vi "S4GUI_001.vi"() -> ()   [LabVIEW 2018] (continued)
                    n596 = stacked-sequence "Atualizacao dos indicadores inferiores do CANAL C da tela principal" {
                      tunnel: w1340 -> [w1355 w1358 w1363 w1372 w1375 w1379]
                      tunnel: [w1341 _ _ _ _ _] -> w1339
                      tunnel: [_ w1356 _ _ _ _] -> w1338
                      tunnel: [_ _ w1361 _ _ _] -> w1337
                      tunnel: [_ _ _ w1366 _ _] -> w1336
                      tunnel: [_ _ _ _ w1373 _] -> w1335
                      tunnel: [_ _ _ _ _ w1376] -> w1334
                      frame #0 {
                        # "SubImage"
                        n597 = Unbundle By Name(w1355) -> ("INITIAL_LINE"=w1353:u16, "FINAL_LINE"=w1352:u16, "INITIAL_COLUMN"=w1351:u16, "FINAL_COLUMN"=w1350:u16)
                        n598 = Number To Decimal String(number=w1353) -> (decimal integer string=w1349:string)  [unwired: 1 in]
                        n599 = Number To Decimal String(number=w1352) -> (decimal integer string=w1347:string)  [unwired: 1 in]
                        n600 = Number To Decimal String(number=w1351) -> (decimal integer string=w1345:string)  [unwired: 1 in]
                        n601 = Number To Decimal String(number=w1350) -> (decimal integer string=w1343:string)  [unwired: 1 in]
                        n602 = Concatenate Strings("[", w1349, ":", w1347, ",", w1345, ":", w1343, "]") -> (w1341:string)
                      }
                      frame #1 {
                        # "Em Active"
                        n603 = Unbundle By Name(w1358) -> ("EM_MODE"=w1357:u8)
                        n604 = case shown="0, Default" w1357 {
                          tunnel: ["Electron M." ("EmActive1") "Convent." ("EmActive1")] -> w1356
                          frame 0, Default {
                          }
                          frame 1 {
                          }
                        }
                      }
                      frame #2 {
                        # "Pre Amp"
                        n605 = Unbundle By Name(w1363) -> ("PREAMP"=w1362:u8)
                        n606 = case shown="1" w1362 {
                          tunnel: ["Gain 1" ("EmActive1") "Gain 2" ("EmActive1")] -> w1361
                          frame 0, Default {
                          }
                          frame 1 {
                          }
                        }
                      }
                      frame #3 {
                        # "Binning"
                        n607 = Unbundle By Name(w1372) -> ("VBIN"=w1371:u16, "HBIN"=w1370:u16)
                        n608 = Number To Decimal String(number=w1370) -> (decimal integer string=w1367:string)  [unwired: 1 in]
                        n609 = Number To Decimal String(number=w1371) -> (decimal integer string=w1369:string)  [unwired: 1 in]
                        n610 = Concatenate Strings(w1369, "x", w1367) -> (w1366:string)
                      }
                      frame #4 {
                        # "Gain"
                        n611 = Unbundle By Name(w1375) -> ("EM_GAIN"=w1374:u16)
                        n612 = Number To Decimal String(number=w1374) -> (decimal integer string=w1373:string)  [unwired: 1 in]
                      }
                      frame #5 {
                        # "Readout"
                        n613 = Unbundle By Name(w1379) -> ("EM_MODE"=w1378:u8, "READOUT_RATE"=w1377:u8)
                        n614 = case shown="0, Default" w1378 {
                          tunnel: w1377 -> [w1381 w1387]
                          tunnel: [w1380 w1386] -> w1376
                          frame 0, Default {
                            n615 = case shown="0, Default" w1381 {
                              tunnel: ["30 MHz" ("EmActive1") "20 MHz" ("EmActive1") "10 MHz" ("EmActive1") "1 MHz" ("EmActive1")] -> w1380
                              frame 0, Default {
                              }
                              frame 1 {
                              }
                              frame 2 {
                              }
                              frame 3 {
                              }
                            }
                          }
                          frame 1 {
                            n616 = case shown="1" w1387 {
                              tunnel: ["1 MHz" ("EmActive1") "0.1 MHz" ("EmActive1")] -> w1386
                              frame 0, Default {
                              }
                              frame 1 {
                              }
                            }
                          }
                        }
                      }
                    }
                  }
                }
                n617 = Unbundle By Name(w1264) -> ("INITIAL_LINE"=w1269:u16, "INITIAL_COLUMN"=w1267:u16, "FINAL_LINE"=w1270:u16, "FINAL_COLUMN"=w1268:u16, "VBIN"=w1273:u16, "HBIN"=w1329:u16, "PREAMP"=w1272:u8, "EM_GAIN"=w1271:u16, "READOUT_RATE"=w1266:u8, "SHUTTER_OPENNING_TIME"=w1328:u16, "SHUTTER_CLOSING_TIME"=w1327:u16, "VERTICAL_SHIFT_SPEED"=w1326:u8, "READ_MODE"=w1325:u8, "VERTICAL_CLOCK_VOLTAGE"=w1324:u8, "AD_CHANNEL"=w1323:u32, "SHUTTER_MODE"=w1318:u8, "SHUTTER_TTL"=w1319:u8, "TRIGGER_MODE"=w1320:u8, "FRAME_TRANSFER"=w1321:bool, "ACQUISITION_MODE"=w1322:u8, "EM_MODE"=w1265:u8)
                n618 = Not(x=w1292) -> (.not. x?=w1312:bool)
                n619 = Not(x=w1291) -> (.not. x?=w1310:bool)
                n620 = Not(x=w1290) -> (.not. x?=w1311:bool)
                n621 = Not(x=w1289) -> (.not. x?=w1309:bool)
                n622 = Not(x=w1295) -> (.not. x?=w1314:bool)
                n623 = Not(x=w1294) -> (.not. x?=w1313:bool)
                n624 = Not(x=w1293) -> (.not. x?=w1315:bool)
                n625 = property on="Image FInal Column 3" class="DigNum (strict)"("Blinking"=w1312) -> ()  [unwired: 2 in, 2 out]
                n626 = property on="Frame Transfer 3" class="Bool (strict)"("Blinking"=w1310) -> ()  [unwired: 2 in, 2 out]
                n627 = property on="Vertical Clock Voltage 3" class="Ring (strict)"("Blinking"=w1311) -> ()  [unwired: 2 in, 2 out]
                n628 = property on="A/D Channel 3" class="DigNum (strict)"("Blinking"=w1309) -> ()  [unwired: 2 in, 2 out]
                n629 = property on="Image Initial Line 3" class="DigNum (strict)"("Blinking"=w1314) -> ()  [unwired: 2 in, 2 out]
                n630 = property on="Image Initial Column 3" class="DigNum (strict)"("Blinking"=w1313) -> ()  [unwired: 2 in, 2 out]
                n631 = property on="Image Final Line 3" class="DigNum (strict)"("Blinking"=w1315) -> ()  [unwired: 2 in, 2 out]
                n632 = Not(x=w1284) -> (.not. x?=w1305:bool)
                n633 = Not(x=w1283) -> (.not. x?=w1307:bool)
                n634 = Not(x=w1282) -> (.not. x?=w1306:bool)
                n635 = Not(x=w1281) -> (.not. x?=w1308:bool)
                n636 = Not(x=w1288) -> (.not. x?=w1304:bool)
                n637 = Not(x=w1287) -> (.not. x?=w1286:bool)
                n638 = Not(x=w1285) -> (.not. x?=w1303:bool)
                n639 = property on="Shutter Openning Time 3" class="DigNum (strict)"("Blinking"=w1305) -> ()  [unwired: 2 in, 2 out]
                n640 = property on="Shutter Closing Time 3" class="DigNum (strict)"("Blinking"=w1307) -> ()  [unwired: 2 in, 2 out]
                n641 = property on="Vertical Binning 3" class="DigNum (strict)"("Blinking"=w1306) -> ()  [unwired: 2 in, 2 out]
                n642 = property on="Horizontal Binning 3" class="DigNum (strict)"("Blinking"=w1308) -> ()  [unwired: 2 in, 2 out]
                n643 = property on="CCD EM Gain 3" class="DigNum (strict)"("Blinking"=w1304) -> ()  [unwired: 2 in, 2 out]
                n644 = property on="Shutter Mode 3" class="Ring (strict)"("Blinking"=w1286) -> ()  [unwired: 2 in, 2 out]
                n645 = property on="Shutter TTL 3" class="Ring (strict)"("Blinking"=w1303) -> ()  [unwired: 2 in, 2 out]
                n646 = local read "Cameras Cluster"() -> (w1331:T5)
                n647 = Bundle By Name(cluster=w1331, "Current Configuration.Image Initial Line 3"=w1269, "Current Configuration.Image Initial Column 3"=w1267, "Current Configuration.Image Final Line 3"=w1270, "Current Configuration.Image FInal Column 3"=w1268, "Current Configuration.Vertical Binning 3"=w1273, "Current Configuration.Horizontal Binning 3"=w1329, "Current Configuration.Pre-amplification Gain 3"=w1272, "Current Configuration.CCD EM Gain 3"=w1271, "Current Configuration.Readout Rate 3"=w1266, "Current Configuration.Shutter Openning Time 3"=w1328, "Current Configuration.Shutter Closing Time 3"=w1327, "Current Configuration.Vertical Shift Speed 3"=w1326, "Current Configuration.Read Mode 3"=w1325, "Current Configuration.Vertical Clock Voltage 3"=w1324, "Current Configuration.A/D Channel 3"=w1323, "Current Configuration.Shutter Mode 3"=w1318, "Current Configuration.Shutter TTL 3"=w1319, "Current Configuration.Trigger Mode 3"=w1320, "Current Configuration.Frame Transfer 3"=w1321, "Current Configuration.Acquisition Mode 3"=w1322, "Current Configuration.CCD EM Mode 3"=w1265) -> (w1330:T5)
                n648 = Not(x=w1280) -> (.not. x?=w1296:bool)
                n649 = Not(x=w1276) -> (.not. x?=w1299:bool)
                n650 = Not(x=w1275) -> (.not. x?=w1297:bool)
                n651 = Not(x=w1274) -> (.not. x?=w1298:bool)
                n652 = Not(x=w1279) -> (.not. x?=w1301:bool)
                n653 = Not(x=w1278) -> (.not. x?=w1300:bool)
                n654 = Not(x=w1277) -> (.not. x?=w1302:bool)
                n655 = local write "RO3"(w1258) -> ()
                n656 = local write "B3"(w1260) -> ()
                n657 = local write "PA3"(w1261) -> ()
                n658 = local write "EA3"(w1262) -> ()
                n659 = local write "G3"(w1259) -> ()
                n660 = local write "SI3"(w1263) -> ()
                n661 = property on="Acquisition Mode 3" class="Ring (strict)"("Blinking"=w1296) -> ()  [unwired: 2 in, 2 out]
                n662 = property on="Readout Rate 3" class="Ring (strict)"("Blinking"=w1299) -> ()  [unwired: 2 in, 2 out]
                n663 = property on="Vertical Shift Speed 3" class="Ring (strict)"("Blinking"=w1297) -> ()  [unwired: 2 in, 2 out]
                n664 = property on="CCD EM Mode 3" class="Ring (strict)"("Blinking"=w1298) -> ()  [unwired: 2 in, 2 out]
                n665 = property on="Trigger Mode 3" class="Ring (strict)"("Blinking"=w1301) -> ()  [unwired: 2 in, 2 out]
                n666 = property on="Read Mode 3" class="Ring (strict)"("Blinking"=w1300) -> ()  [unwired: 2 in, 2 out]
                n667 = property on="Pre-amplification Gain 3" class="Ring (strict)"("Blinking"=w1302) -> ()  [unwired: 2 in, 2 out]
                n668 = local write "Cameras Cluster"(w1330) -> ()
                n669 = Compound Arithmetic op=AND(w1280, w1279, w1278, w1277, w1276, w1275, w1274, w1288, w1287, w1285, w1284, w1283, w1282, w1281, w1295, w1294, w1293, w1292, w1291, w1290, w1289) -> (→"CCD checked 3":bool)
              }
              frame #18 {
                # "Carrega coluna do Channel 4"
                # "Aba:  Eng->Camera"
                n670 = Unbundle By Name(w1465) -> ("ChannelD_CCD"=w1397:T21, "CHD_Checked Params"=w1450:T22, "ChannelD_Status.connection"=w1396:bool)
                n671 = Unbundle By Name(w1450) -> ("ACQUISITION_MODE"=w1414:bool, "TRIGGER_MODE"=w1413:bool, "READ_MODE"=w1412:bool, "PREAMP"=w1410:bool, "READOUT_RATE"=w1409:bool, "VERTICAL_SHIFT_SPEED"=w1408:bool, "EM_MODE"=w1407:bool, "EM_GAIN"=w1421:bool, "SHUTTER_MODE"=w1420:bool, "SHUTTER_TTL"=w1419:bool, "SHUTTER_OPENING_TIME"=w1418:bool, "SHUTTER_CLOSING_TIME"=w1417:bool, "VBIN"=w1416:bool, "HBIN"=w1415:bool, "INITIAL_LINE"=w1428:bool, "INITIAL_COLUMN"=w1427:bool, "FINAL_LINE"=w1426:bool, "FINAL_COLUMN"=w1425:bool, "FRAME_TRANSFER"=w1424:bool, "VERTICAL_CLOCK_VOLTAGE"=w1423:bool, "AD_CHANNEL"=w1422:bool)
                n672 = case shown="False" w1396 {
                  tunnel: w1397 -> [_ w1473]
                  tunnel: [w1466 w1472] -> w1395
                  tunnel: [w1466 w1471] -> w1394
                  tunnel: [w1466 w1470] -> w1393
                  tunnel: [w1466 w1469] -> w1392
                  tunnel: [w1466 w1468] -> w1391
                  tunnel: [w1466 w1467] -> w1390
                  frame False {
                    w1466 = ""
                  }
                  frame True {
                    n673 = stacked-sequence "Atualizacao dos indicadores inferiores do CANAL D da tela principal" {
                      tunnel: w1473 -> [w1488 w1491 w1496 w1505 w1508 w1512]
                      tunnel: [w1474 _ _ _ _ _] -> w1472
                      tunnel: [_ w1489 _ _ _ _] -> w1471
                      tunnel: [_ _ w1494 _ _ _] -> w1470
                      tunnel: [_ _ _ w1499 _ _] -> w1469
                      tunnel: [_ _ _ _ w1506 _] -> w1468
                      tunnel: [_ _ _ _ _ w1509] -> w1467
                      frame #0 {
                        # "SubImage"
                        n674 = Unbundle By Name(w1488) -> ("INITIAL_LINE"=w1486:u16, "FINAL_LINE"=w1485:u16, "INITIAL_COLUMN"=w1484:u16, "FINAL_COLUMN"=w1483:u16)
                        n675 = Number To Decimal String(number=w1486) -> (decimal integer string=w1482:string)  [unwired: 1 in]
                        n676 = Number To Decimal String(number=w1485) -> (decimal integer string=w1480:string)  [unwired: 1 in]
                        n677 = Number To Decimal String(number=w1484) -> (decimal integer string=w1478:string)  [unwired: 1 in]
                        n678 = Number To Decimal String(number=w1483) -> (decimal integer string=w1476:string)  [unwired: 1 in]
                        n679 = Concatenate Strings("[", w1482, ":", w1480, ",", w1478, ":", w1476, "]") -> (w1474:string)
                      }
                      frame #1 {
                        # "Em Active"
                        n680 = Unbundle By Name(w1491) -> ("EM_MODE"=w1490:u8)
                        n681 = case shown="0, Default" w1490 {
                          tunnel: ["Electron M." ("EmActive1") "Convent." ("EmActive1")] -> w1489
                          frame 0, Default {
                          }
                          frame 1 {
                          }
                        }
                      }
                      frame #2 {
                        # "Pre Amp"
                        n682 = Unbundle By Name(w1496) -> ("PREAMP"=w1495:u8)
                        n683 = case shown="1" w1495 {
                          tunnel: ["Gain 1" ("EmActive1") "Gain 2" ("EmActive1")] -> w1494
                          frame 0, Default {
                          }
                          frame 1 {
                          }
                        }
                      }
                      frame #3 {
                        # "Binning"
                        n684 = Unbundle By Name(w1505) -> ("VBIN"=w1504:u16, "HBIN"=w1503:u16)
                        n685 = Number To Decimal String(number=w1503) -> (decimal integer string=w1500:string)  [unwired: 1 in]
                        n686 = Number To Decimal String(number=w1504) -> (decimal integer string=w1502:string)  [unwired: 1 in]
                        n687 = Concatenate Strings(w1502, "x", w1500) -> (w1499:string)
                      }
                      frame #4 {
                        # "Gain"
                        n688 = Unbundle By Name(w1508) -> ("EM_GAIN"=w1507:u16)
                        n689 = Number To Decimal String(number=w1507) -> (decimal integer string=w1506:string)  [unwired: 1 in]
                      }
                      frame #5 {
                        # "Readout"
                        n690 = Unbundle By Name(w1512) -> ("EM_MODE"=w1511:u8, "READOUT_RATE"=w1510:u8)
                        n691 = case shown="0, Default" w1511 {
                          tunnel: w1510 -> [w1514 w1520]
                          tunnel: [w1513 w1519] -> w1509
                          frame 0, Default {
                            n692 = case shown="0, Default" w1514 {
                              tunnel: ["30 MHz" ("EmActive1") "20 MHz" ("EmActive1") "10 MHz" ("EmActive1") "1 MHz" ("EmActive1")] -> w1513
                              frame 0, Default {
                              }
                              frame 1 {
                              }
                              frame 2 {
                              }
                              frame 3 {
                              }
                            }
                          }
                          frame 1 {
                            n693 = case shown="1" w1520 {
                              tunnel: ["1 MHz" ("EmActive1") "0.1 MHz" ("EmActive1")] -> w1519
                              frame 0, Default {
                              }
                              frame 1 {
                              }
                            }
                          }
                        }
                      }
                    }
                  }
                }
                n694 = Unbundle By Name(w1397) -> ("INITIAL_LINE"=w1402:u16, "INITIAL_COLUMN"=w1400:u16, "FINAL_LINE"=w1403:u16, "FINAL_COLUMN"=w1401:u16, "VBIN"=w1406:u16, "HBIN"=w1462:u16, "PREAMP"=w1405:u8, "EM_GAIN"=w1404:u16, "READOUT_RATE"=w1399:u8, "SHUTTER_OPENNING_TIME"=w1461:u16, "SHUTTER_CLOSING_TIME"=w1460:u16, "VERTICAL_SHIFT_SPEED"=w1459:u8, "READ_MODE"=w1458:u8, "VERTICAL_CLOCK_VOLTAGE"=w1457:u8, "AD_CHANNEL"=w1456:u32, "SHUTTER_MODE"=w1451:u8, "SHUTTER_TTL"=w1452:u8, "TRIGGER_MODE"=w1453:u8, "FRAME_TRANSFER"=w1454:bool, "ACQUISITION_MODE"=w1455:u8, "EM_MODE"=w1398:u8)
                n695 = Not(x=w1425) -> (.not. x?=w1445:bool)
                n696 = Not(x=w1424) -> (.not. x?=w1443:bool)
                n697 = Not(x=w1423) -> (.not. x?=w1444:bool)
                n698 = Not(x=w1422) -> (.not. x?=w1442:bool)
                n699 = Not(x=w1428) -> (.not. x?=w1447:bool)
                n700 = Not(x=w1427) -> (.not. x?=w1446:bool)
                n701 = Not(x=w1426) -> (.not. x?=w1448:bool)
                n702 = property on="Image FInal Column 4" class="DigNum (strict)"("Blinking"=w1445) -> ()  [unwired: 2 in, 2 out]
                n703 = property on="Frame Transfer 4" class="Bool (strict)"("Blinking"=w1443) -> ()  [unwired: 2 in, 2 out]
                n704 = property on="Vertical Clock Voltage 4" class="Ring (strict)"("Blinking"=w1444) -> ()  [unwired: 2 in, 2 out]
                n705 = property on="A/D Channel 4" class="DigNum (strict)"("Blinking"=w1442) -> ()  [unwired: 2 in, 2 out]
                n706 = property on="Image Initial Line 4" class="DigNum (strict)"("Blinking"=w1447) -> ()  [unwired: 2 in, 2 out]
                n707 = property on="Image Initial Column 4" class="DigNum (strict)"("Blinking"=w1446) -> ()  [unwired: 2 in, 2 out]
                n708 = property on="Image Final Line 4" class="DigNum (strict)"("Blinking"=w1448) -> ()  [unwired: 2 in, 2 out]
                n709 = Not(x=w1418) -> (.not. x?=w1438:bool)
                n710 = Not(x=w1417) -> (.not. x?=w1440:bool)
                n711 = Not(x=w1416) -> (.not. x?=w1439:bool)
                n712 = Not(x=w1415) -> (.not. x?=w1441:bool)
                n713 = Not(x=w1421) -> (.not. x?=w1436:bool)
                n714 = Not(x=w1420) -> (.not. x?=w1437:bool)
                n715 = Not(x=w1419) -> (.not. x?=w1435:bool)
                n716 = property on="Shutter Openning Time 4" class="DigNum (strict)"("Blinking"=w1438) -> ()  [unwired: 2 in, 2 out]
                n717 = property on="Shutter Closing Time 4" class="DigNum (strict)"("Blinking"=w1440) -> ()  [unwired: 2 in, 2 out]
                n718 = property on="Vertical Binning 4" class="DigNum (strict)"("Blinking"=w1439) -> ()  [unwired: 2 in, 2 out]
                n719 = property on="Horizontal Binning 4" class="DigNum (strict)"("Blinking"=w1441) -> ()  [unwired: 2 in, 2 out]
                n720 = property on="CCD EM Gain 4" class="DigNum (strict)"("Blinking"=w1436) -> ()  [unwired: 2 in, 2 out]
                n721 = property on="Shutter Mode 4" class="Ring (strict)"("Blinking"=w1437) -> ()  [unwired: 2 in, 2 out]
                n722 = property on="Shutter TTL 4" class="Ring (strict)"("Blinking"=w1435) -> ()  [unwired: 2 in, 2 out]
                n723 = local read "Cameras Cluster"() -> (w1464:T5)
                n724 = Bundle By Name(cluster=w1464, "Current Configuration.Image Initial Line 4"=w1402, "Current Configuration.Image Initial Column 4"=w1400, "Current Configuration.Image Final Line 4"=w1403, "Current Configuration.Image FInal Column 4"=w1401, "Current Configuration.Vertical Binning 4"=w1406, "Current Configuration.Horizontal Binning 4"=w1462, "Current Configuration.Pre-amplification Gain 4"=w1405, "Current Configuration.CCD EM Gain 4"=w1404, "Current Configuration.Readout Rate 4"=w1399, "Current Configuration.Shutter Openning Time 4"=w1461, "Current Configuration.Shutter Closing Time 4"=w1460, "Current Configuration.Vertical Shift Speed 4"=w1459, "Current Configuration.Read Mode 4"=w1458, "Current Configuration.Vertical Clock Voltage 4"=w1457, "Current Configuration.A/D Channel 4"=w1456, "Current Configuration.Shutter Mode 4"=w1451, "Current Configuration.Shutter TTL 4"=w1452, "Current Configuration.Trigger Mode 4"=w1453, "Current Configuration.Frame Transfer 4"=w1454, "Current Configuration.Acquisition Mode 4"=w1455, "Current Configuration.CCD EM Mode 4"=w1398) -> (w1463:T5)
                n725 = local write "SI4"(w1395) -> ()
                n726 = local write "RO4"(w1390) -> ()
                n727 = local write "PA4"(w1393) -> ()
                n728 = local write "EA4"(w1394) -> ()
                n729 = local write "G4"(w1391) -> ()
                n730 = local write "B4"(w1392) -> ()
                n731 = Not(x=w1414) -> (.not. x?=w1429:bool)
                n732 = Not(x=w1409) -> (.not. x?=w1432:bool)
                n733 = Not(x=w1408) -> (.not. x?=w1430:bool)
                n734 = Not(x=w1407) -> (.not. x?=w1431:bool)
                n735 = Not(x=w1413) -> (.not. x?=w1433:bool)
                n736 = Not(x=w1412) -> (.not. x?=w1411:bool)
                n737 = Not(x=w1410) -> (.not. x?=w1434:bool)
                n738 = property on="Acquisition Mode 4" class="Ring (strict)"("Blinking"=w1429) -> ()  [unwired: 2 in, 2 out]
                n739 = property on="Readout Rate 4" class="Ring (strict)"("Blinking"=w1432) -> ()  [unwired: 2 in, 2 out]
                n740 = property on="Vertical Shift Speed 4" class="Ring (strict)"("Blinking"=w1430) -> ()  [unwired: 2 in, 2 out]
                n741 = property on="CCD EM Mode 4" class="Ring (strict)"("Blinking"=w1431) -> ()  [unwired: 2 in, 2 out]
                n742 = property on="Trigger Mode 4" class="Ring (strict)"("Blinking"=w1433) -> ()  [unwired: 2 in, 2 out]
                n743 = property on="Read Mode 4" class="Ring (strict)"("Blinking"=w1411) -> ()  [unwired: 2 in, 2 out]
                n744 = property on="Pre-amplification Gain 4" class="Ring (strict)"("Blinking"=w1434) -> ()  [unwired: 2 in, 2 out]
                n745 = local write "Cameras Cluster"(w1463) -> ()
                n746 = Compound Arithmetic op=AND(w1414, w1413, w1412, w1410, w1409, w1408, w1407, w1421, w1420, w1419, w1418, w1417, w1416, w1415, w1428, w1427, w1426, w1425, w1424, w1423, w1422) -> (→"CCD checked 4":bool)
              }
            }
            n747 = stacked-sequence {
              tunnel: w179 -> [w191 w195 w203 w210 w224]
              tunnel: w178 -> [w190 w194 w202 w209 w223]
              tunnel: [_ _ _ _ w215] -> w170
              tunnel: [_ _ _ _ w216] -> w169
              frame #0 {
                n748 = call-dynamic "Read AcquisitionA.vi"("error in (no error)"=w190, "S4ACS_GUI in"=w191) -> ("error out"=w187:errorcluster, "Acquisition.lvclass"=w189:refnum<class "Acquisition.lvclass">)  [unwired: 7 in, 1 out]
                n749 = call-dynamic "Read Channel.vi"("error in (no error)"=w187, "Acquisition in"=w189) -> ("error out"=w186:errorcluster, "Channel.lvclass"=w188:refnum<class "Channel.lvclass">)  [unwired: 7 in, 1 out]
                n750 = call-dynamic "Read CyclesDone.vi"("error in (no error)"=w186, "Channel in"=w188) -> ("error out"=→"error out 6":errorcluster, "CyclesDone"=→"Cycles Done ch1":u32)  [unwired: 7 in, 1 out]
              }
              frame #1 {
                n751 = call "Read AcquisitionB.vi"("error in (no error)"=w194, "S4ACS_GUI in"=w195) -> ("error out"=w197:errorcluster, "Acquisition.lvclass"=w198:refnum<class "Acquisition.lvclass">)  [unwired: 7 in, 1 out]
                n752 = call-dynamic "Read Channel.vi"("error in (no error)"=w197, "Acquisition in"=w198) -> ("error out"=w196:errorcluster, "Channel.lvclass"=w199:refnum<class "Channel.lvclass">)  [unwired: 7 in, 1 out]
                n753 = call-dynamic "Read CyclesDone.vi"("error in (no error)"=w196, "Channel in"=w199) -> ("error out"=→"error out 4":errorcluster, "CyclesDone"=→"Cycles Done ch2":u32)  [unwired: 7 in, 1 out]
              }
              frame #2 {
                n754 = call-dynamic "Read AcquisitionC.vi"("error in (no error)"=w202, "S4ACS_GUI in"=w203) -> ("error out"=w205:errorcluster, "Acquisition.lvclass"=w206:refnum<class "Acquisition.lvclass">)  [unwired: 7 in, 1 out]
                n755 = call-dynamic "Read Channel.vi"("error in (no error)"=w205, "Acquisition in"=w206) -> ("error out"=w204:errorcluster, "Channel.lvclass"=w207:refnum<class "Channel.lvclass">)  [unwired: 7 in, 1 out]
                n756 = call-dynamic "Read CyclesDone.vi"("error in (no error)"=w204, "Channel in"=w207) -> ("error out"=→"error out 5":errorcluster, "CyclesDone"=→"Cycles Done ch3":u32)  [unwired: 7 in, 1 out]
              }
              frame #3 {
                n757 = call-dynamic "Read AcquisitionD.vi"("error in (no error)"=w209, "S4ACS_GUI in"=w210) -> ("error out"=w212:errorcluster, "Acquisition.lvclass"=w213:refnum<class "Acquisition.lvclass">)  [unwired: 7 in, 1 out]
                n758 = call-dynamic "Read Channel.vi"("error in (no error)"=w212, "Acquisition in"=w213) -> ("error out"=w211:errorcluster, "Channel.lvclass"=w214:refnum<class "Channel.lvclass">)  [unwired: 7 in, 1 out]
                n759 = call-dynamic "Read CyclesDone.vi"("error in (no error)"=w211, "Channel in"=w214) -> ("CyclesDone"=→"Cycles Done ch4":u32)  [unwired: 7 in, 2 out]
              }
              frame #4 {
                (unwired) cluster{"AG status":bool, "rotator":dbl} {"AG status"=FALSE, "rotator"=0.0} ("element")
                n760 = call-dynamic "Read guider queue.vi"("error in (no error)"=w223, "S4GUI in"=w224) -> ("error out"=w218:errorcluster, "guider queue"=w222:refnum<queue>, "S4GUI out"=w217:refnum<class "S4GUI.lvclass">)  [unwired: 7 in]
                n761 = Get Queue Status(queue=w222, error in (no error)=w218) -> (queue out=w220:refnum<queue>, error out=w219:errorcluster, # elements in queue=w221:i32)  [unwired: 1 in, 5 out]
                n762 = case shown="Default" w221 {
                  tunnel: w220 -> [_ w237]
                  tunnel: w219 -> [w225 w236]
                  tunnel: w217 -> [w226 w231]
                  tunnel: [w225 w229] -> w216
                  tunnel: [w226 w230] -> w215
                  frame 0 {
                  }
                  frame Default {
                    n763 = Dequeue Element(queue=w237, error in (no error)=w236) -> (queue out=w234:refnum<queue>, element=w233:cluster{"AG status":bool, "rotator":dbl}, error out=w235:errorcluster)  [unwired: 1 in, 1 out]
                    n764 = Unbundle By Name(w233) -> ("AG status"=→"GUIDER":bool, "rotator"=w227:dbl)
                    "rotator" <- w227
                    n765 = Flush Queue(queue=w234, error in (no error)=w235) -> (error out=w228:errorcluster)  [unwired: 2 out]
                    n766 = call-dynamic "Write rotator.vi"("error in (no error)"=w228, "rotator"=w227, "S4GUI in"=w231) -> ("error out"=w229:errorcluster, "S4GUI out"=w230:refnum<class "S4GUI.lvclass">)  [unwired: 7 in]
                  }
                }
              }
            }
            n767 = call-dynamic "Read Obs_state.vi"("error in (no error)"=w169, "S4ACS_GUI in"=w170) -> ("error out"=w165:errorcluster, "Obs_state"=w166:u32, "S4ACS_GUI out"=w164:refnum<class "S4GUI.lvclass">)  [unwired: 7 in]
            n768 = In Range and Coerce(upper limit=u32 226, x=w166, lower limit=u32 220 ("upper limit")) -> (In Range?=w162:bool)  [unwired: 1 out]
            n769 = Select(t="STOP", s=w162, f="INIT") -> (s? t:f=w161:string)
            n770 = property on="Init mode" class="Bool"(error in=w165, "Blinking"=w162, "Caption.Visible"=w162, "BoolText.Text"=w161) -> (error out=w163:errorcluster)  [unwired: 1 in, 1 out]
            n771 = call-dynamic "Read cyclesDone.vi"("error in (no error)"=w163, "S4GUI in"=w164) -> ("error out"=w154:errorcluster, "cyclesDone"=→"#Cycles Done":u32, "S4GUI out"=w156:refnum<class "S4GUI.lvclass">)  [unwired: 7 in]
            n772 = call-dynamic "Read cycles wprot.vi"("error in (no error)"=w154, "S4GUI in"=w156) -> ("cycles wprot"=→"Cycles Counter":u32)  [unwired: 7 in, 2 out]
            n773 = call "Read Instrument.lvclass.vi"("error in (no error)"=w154, "S4ACS_GUI in"=w156) -> ("error out"=w175:errorcluster, "Instrument.lvclass"=w172:refnum<class "Instrument.lvclass">, "S4ACS_GUI out"=w177:refnum<class "S4GUI.lvclass">)  [unwired: 7 in]
            n774 = call-dynamic "Write mode.vi"("error in (no error)"=w175, "mode"=w157, "Instrument in"=w172) -> ("error out"=w174:errorcluster, "Instrument out"=w171:refnum<class "Instrument.lvclass">)  [unwired: 7 in]
            n775 = call "Write Instrument.lvclass.vi"("error in (no error)"=w174, "Instrument.lvclass"=w171, "S4ACS_GUI in"=w177) -> ("error out"=w173:errorcluster, "S4ACS_GUI out"=w176:refnum<class "S4GUI.lvclass">)  [unwired: 7 in]
          }
        }
        n776 = Or(x="stop", y="stop 2") -> (x .or. y?=w134:bool)
      }
      event "TCS mode": Value Change {
        # "simul"
        # "real"
        # "Inicializar nova comunicação, de acordo\n com valor de TCSmode\n\nServer.Write id (T=8 ou F=9)\nTCS.Init"
        # "Parar a comunciação atual\nServer.End"
        n777 = event-data() -> ("NewVal"=w1525:bool)  [unwired: 1 in, 5 out]
        n778 = call-dynamic "Read TCS.lvclass.vi"("error in (no error)"=w1535, "S4GUI in"=w1536) -> ("error out"=w1530:errorcluster, "TCS.lvclass"=w1533:refnum<class "TCS.lvclass">, "S4GUI out"=w1534:refnum<class "S4GUI.lvclass">)  [unwired: 7 in]
        n779 = call-dynamic "End.vi"("error in (no error)"=w1530, "Server in"=w1533) -> ("error out"=w1529:errorcluster, "Server out"=w1532:refnum<class "TCS.lvclass">)  [unwired: 8 in]
        n780 = Select(t=u32 8, s=w1525, f=u32 9) -> (s? t:f=w1539:u32)
        n781 = call-dynamic "Write id.vi"("error in (no error)"=w1529, "id"=w1539, "Server in"=w1532) -> ("error out"=w1528:errorcluster, "Server out"=w1531:refnum<class "TCS.lvclass">)  [unwired: 7 in]
        n782 = call-dynamic "Initialize.vi"("error in (no error)"=w1528, "TCS in"=w1531) -> ("error out"=w1526:errorcluster, "TCS out"=w1527:refnum<class "TCS.lvclass">)  [unwired: 8 in]
        n783 = call-dynamic "Write TCS.lvclass.vi"("error in (no error)"=w1526, "TCS.lvclass"=w1527, "S4GUI in"=w1534) -> ("error out"=w1523:errorcluster, "S4GUI out"=w1524:refnum<class "S4GUI.lvclass">)  [unwired: 7 in]
      }
      event "Set from Input ch1": Value Change {
        # "ACS"
        # "GUI"
        # "EM_MODE = E.M."
        # "Readou Rate:\n30         0\n20         1     \n10         2\n1           3"
        # "EM_MODE = Conv"
        # "Readou Rate:\n1         0\n0.1      1"
        # "Readou Rate:\n1         0\n0.1      1     \n10       2\n20       3\n30       4"
        n784 = event-data() -> ()  [unwired: 1 in, 6 out]
        n785 = local read "Input Cluster"() -> (w1555:T6)
        n786 = Unbundle By Name(w1555) -> ("Parameters"=w1554:T23)
        n787 = Unbundle By Name(w1554) -> ("Image \nInitial Line"=w1582:u16, "Image\nInitial Column"=w1581:u16, "Image\nFinal Line"=w1580:u16, "Image\nFInal Column"=w1579:u16, "Vertical\nBinning"=w1578:u16, "Horizontal\nBinning"=w1577:u16, "Pre-amplification\nGain"=w1576:u8, "CCD\nEM Gain"=w1575:u16, "Readout\nRate"=w1574:u8, "Shutter\nOpenning Time"=w1573:i32, "Shutter\nClosing Time"=w1572:i32, "Vertical\nShift Speed"=w1571:u8, "Read\nMode"=w1570:u8, "Vertical\nClock Voltage"=w1569:u8, "A/D \nChannel"=w1568:u32, "Shutter\nMode"=w1567:u16, "Shutter\nTTL"=w1566:u16, "Trigger\nMode"=w1565:u16, "Frame\nTransfer"=w1543:bool, "Acquisition\nMode"=w1564:u8, "CCD \nEM Mode"=w1563:u8)
        n788 = call-dynamic "Read AcquisitionA.vi"("error in (no error)"=w1546, "S4ACS_GUI in"=w1547) -> ("error out"=w1603:errorcluster, "Acquisition.lvclass"=w1607:refnum<class "Acquisition.lvclass">, "S4ACS_GUI out"=w1608:refnum<class "S4GUI.lvclass">)  [unwired: 7 in]
        n789 = call-dynamic "Read Channel.vi"("error in (no error)"=w1603, "Acquisition in"=w1607) -> ("error out"=w1602:errorcluster, "Channel.lvclass"=w1605:refnum<class "Channel.lvclass">, "Acquisition out"=w1606:refnum<class "Acquisition.lvclass">)  [unwired: 7 in]
        n790 = call-dynamic "Read Interface.vi"("error in (no error)"=w1602, "Channel in"=w1605) -> ("error out"=w1542:errorcluster, "Interface.lvclass"=w1544:refnum<class "Interface.lvclass">, "Channel out"=w1604:refnum<class "Channel.lvclass">)  [unwired: 7 in]
        n791 = call-dynamic "Write PREV_FT.vi"("error in (no error)"=w1542, "PREV_FT"=w1543, "Interface in"=w1544) -> ("error out"=w1541:errorcluster, "Interface out"=w1540:refnum<class "Interface.lvclass">)  [unwired: 7 in]
        n792 = call-dynamic "Get CCD_Config.vi"("error in (no error)"=w1541, "Interface in"=w1540) -> ("error out"=w1583:errorcluster, "output cluster"=w1585:T24, "Interface out"=w1584:refnum<class "Interface.lvclass">)  [unwired: 7 in]
        n793 = Bundle By Name(cluster=w1585, "INITIAL_LINE"=w1582, "INITIAL_COLUMN"=w1581, "FINAL_LINE"=w1580, "FINAL_COLUMN"=w1579, "VBIN"=w1578, "HBIN"=w1577, "PREAMP"=w1576, "EM_GAIN"=w1575, "READOUT_RATE"=w1574, "SHUTTER_OPENING_TIME"=w1573, "SHUTTER_CLOSING_TIME"=w1572, "VERTICAL_SHIFT_SPEED"=w1571, "READ_MODE"=w1570, "VERTICAL_CLOCK_VOLTAGE"=w1569, "AD_CHANNEL"=w1568, "SHUTTER_MODE"=w1567, "SHUTTER_TTL"=w1566, "TRIGGER_MODE"=w1565, "FRAME_TRANSFER"=w1543, "ACQUISITION_MODE"=w1564, "EM_MODE"=w1563) -> (w1553:T24)
        n794 = call-dynamic "Set CCD_Config.vi"("error in (no error)"=w1583, "input cluster"=w1553, "Interface in"=w1584) -> ("error out"=w1588:errorcluster, "Interface out"=w1589:refnum<class "Interface.lvclass">)  [unwired: 7 in]
        n795 = Flatten To String(anything=w1553, error in (no error)=w1588) -> (data string=w1591:string, error out=w1590:errorcluster)  [unwired: 2 in, 1 out]
        n796 = call "Write flatted cluster.vi"("error in (no error)"=w1590, "flatted cluster"=w1591, "Interface in"=w1589) -> ("error out"=w1587:errorcluster, "Interface out"=w1586:refnum<class "Interface.lvclass">)  [unwired: 7 in]
        n797 = call-dynamic "Write Interface.vi"("error in (no error)"=w1587, "Interface.lvclass"=w1586, "Channel in"=w1604) -> ("error out"=w1558:errorcluster, "Channel out"=w1561:refnum<class "Channel.lvclass">)  [unwired: 7 in]
        n798 = call "Write section_name.vi"("error in (no error)"=w1558, "section_name"="CCD_ACS1", "Channel in"=w1561) -> ("error out"=w1557:errorcluster, "Channel out"=w1560:refnum<class "Channel.lvclass">)  [unwired: 7 in]
        n799 = call-dynamic "save config.vi"("error in (no error)"=w1557, "file config"="lastsaved.cfg", "Channel in"=w1560) -> ("error out"=w1556:errorcluster, "Channel out"=w1559:refnum<class "Channel.lvclass">)  [unwired: 7 in]
        n800 = call-dynamic "Read State Machine.vi"("error in (no error)"=w1556, "Device in"=w1559) -> ("error out"=w1598:errorcluster, "State Machine.lvclass"=w1600:refnum<class "State Machine.lvclass">, "Device out"=w1601:refnum<class "Channel.lvclass">)  [unwired: 7 in]
        n801 = call-dynamic "Write State.vi"("error in (no error)"=w1598, "State"=60, "State Machine in"=w1600) -> ("error out"=w1597:errorcluster, "State Machine out"=w1599:refnum<class "State Machine.lvclass">)  [unwired: 7 in]
        n802 = call-dynamic "Write State Machine.vi"("error in (no error)"=w1597, "State Machine.lvclass"=w1599, "Device in"=w1601) -> ("error out"=w1594:errorcluster, "Device out"=w1595:refnum<class "Channel.lvclass">)  [unwired: 7 in]
        n803 = call-dynamic "Write Channel.vi"("error in (no error)"=w1594, "Channel.lvclass"=w1595, "Acquisition in"=w1606) -> ("error out"=w1593:errorcluster, "Acquisition out"=w1592:refnum<class "Acquisition.lvclass">)  [unwired: 7 in]
        n804 = call-dynamic "Write AcquisitionA.vi"("error in (no error)"=w1593, "Acquisition.lvclass"=w1592, "S4ACS_GUI in"=w1608) -> ("error out"=w1548:errorcluster, "S4ACS_GUI out"=w1549:refnum<class "S4GUI.lvclass">)  [unwired: 7 in]
        n805 = call "Write cfg file.vi"("error in (no error)"=w1548, "cfg file"="lastsaved.cfg", "S4ACS_GUI in"=w1549) -> ("error out"=w1551:errorcluster, "S4ACS_GUI out"=w1552:refnum<class "S4GUI.lvclass">)  [unwired: 7 in]
      }
      event "Input Cluster.Parameters.CCD \nEM Mode": Value Change {
        n806 = event-data() -> ()  [unwired: 1 in, 6 out]
        n807 = local read "Input Cluster"() -> (w1623:T6)
        n808 = Unbundle By Name(w1623) -> ("Parameters"=w1624:T23)
        n809 = Unbundle By Name(w1624) -> ("Readout\nRate"=→"Readout\nRate":u8, "CCD \nEM Mode"=w1618:u8)
        n810 = case shown="1" w1618 {
          tunnel: [string[] ["30 MHz", "20 MHz", "10 MHz", "1 MHz"] ("Strings []") string[] ["1 MHz", "0.1 MHz"] ("Strings []")] -> w1617
          tunnel: [u8 3 u8 0] -> w1616
          frame 0, Default {
          }
          frame 1 {
          }
        }
        n811 = local read "Cameras Cluster"() -> (w1611:T5)
        n812 = Unbundle By Name(w1611) -> ("Current Configuration"=w1612:T25)
        n813 = flat-sequence {
          tunnel: w1616 -> [w1626]
          tunnel: w1617 -> [w1625]
          tunnel: w1618 -> [w1627]
          tunnel: [w1627] -> w1615
          tunnel: [w1626] -> w1613
          tunnel: w1624 -> [w1633]
          tunnel: [w1632] -> w1622
          tunnel: w1615 -> [w1628]
          tunnel: w1613 -> [w1629]
          tunnel: w1612 -> [w1631]
          tunnel: [w1630] -> w1610
          frame #0 {
            n814 = property on="Readout\nRate" class="Ring (strict)"("Strings []"=w1625) -> ()  [unwired: 2 in, 2 out]
            n815 = property on="Readout Rate" class="Ring (strict)"("Strings []"=w1625) -> ()  [unwired: 2 in, 2 out]
            n816 = property on="Readout Rate 4" class="Ring (strict)"("Strings []"=w1625) -> ()  [unwired: 2 in, 2 out]
            n817 = property on="Readout Rate 2" class="Ring (strict)"("Strings []"=w1625) -> ()  [unwired: 2 in, 2 out]
            n818 = property on="Readout Rate 3" class="Ring (strict)"("Strings []"=w1625) -> ()  [unwired: 2 in, 2 out]
          }
          frame #1 {
            n819 = Bundle By Name(cluster=w1631, "Readout Rate"=w1629, "Read Mode"=w1628) -> (w1630:T25)
            n820 = Bundle By Name(cluster=w1633, "Readout\nRate"=w1629, "CCD \nEM Mode"=w1628) -> (w1632:T23)
          }
        }
        n821 = Bundle By Name(cluster=w1623, "Parameters"=w1622) -> (w1621:T6)
        n822 = Bundle By Name(cluster=w1611, "Current Configuration"=w1610) -> (w1609:T5)
        n823 = local write "Input Cluster"(w1621) -> ()
        n824 = local write "Cameras Cluster"(w1609) -> ()
      }
      event "Set from Input ch2": Value Change {
        n825 = event-data() -> ()  [unwired: 1 in, 6 out]
        n826 = local read "Input Cluster"() -> (w1651:T6)
        n827 = Unbundle By Name(w1651) -> ("Parameters"=w1650:T23)
        n828 = Unbundle By Name(w1650) -> ("Image \nInitial Line"=w1678:u16, "Image\nInitial Column"=w1677:u16, "Image\nFinal Line"=w1676:u16, "Image\nFInal Column"=w1675:u16, "Vertical\nBinning"=w1674:u16, "Horizontal\nBinning"=w1673:u16, "Pre-amplification\nGain"=w1672:u8, "CCD\nEM Gain"=w1671:u16, "Readout\nRate"=w1670:u8, "Shutter\nOpenning Time"=w1669:i32, "Shutter\nClosing Time"=w1668:i32, "Vertical\nShift Speed"=w1667:u8, "Read\nMode"=w1666:u8, "Vertical\nClock Voltage"=w1665:u8, "A/D \nChannel"=w1664:u32, "Shutter\nMode"=w1663:u16, "Shutter\nTTL"=w1662:u16, "Trigger\nMode"=w1661:u16, "Frame\nTransfer"=w1638:bool, "Acquisition\nMode"=w1660:u8, "CCD \nEM Mode"=w1659:u8)
        n829 = call "Read AcquisitionB.vi"("error in (no error)"=w1705, "S4ACS_GUI in"=w1706) -> ("error out"=w1699:errorcluster, "Acquisition.lvclass"=w1703:refnum<class "Acquisition.lvclass">, "S4ACS_GUI out"=w1704:refnum<class "S4GUI.lvclass">)  [unwired: 7 in]
        n830 = call-dynamic "Read Channel.vi"("error in (no error)"=w1699, "Acquisition in"=w1703) -> ("error out"=w1698:errorcluster, "Channel.lvclass"=w1701:refnum<class "Channel.lvclass">, "Acquisition out"=w1702:refnum<class "Acquisition.lvclass">)  [unwired: 7 in]
        n831 = call-dynamic "Read Interface.vi"("error in (no error)"=w1698, "Channel in"=w1701) -> ("error out"=w1641:errorcluster, "Interface.lvclass"=w1642:refnum<class "Interface.lvclass">, "Channel out"=w1700:refnum<class "Channel.lvclass">)  [unwired: 7 in]
        n832 = call-dynamic "Write PREV_FT.vi"("error in (no error)"=w1641, "PREV_FT"=w1638, "Interface in"=w1642) -> ("error out"=w1639:errorcluster, "Interface out"=w1640:refnum<class "Interface.lvclass">)  [unwired: 7 in]
        n833 = call-dynamic "Get CCD_Config.vi"("error in (no error)"=w1639, "Interface in"=w1640) -> ("error out"=w1679:errorcluster, "output cluster"=w1681:T24, "Interface out"=w1680:refnum<class "Interface.lvclass">)  [unwired: 7 in]
        n834 = Bundle By Name(cluster=w1681, "INITIAL_LINE"=w1678, "INITIAL_COLUMN"=w1677, "FINAL_LINE"=w1676, "FINAL_COLUMN"=w1675, "VBIN"=w1674, "HBIN"=w1673, "PREAMP"=w1672, "EM_GAIN"=w1671, "READOUT_RATE"=w1670, "SHUTTER_OPENING_TIME"=w1669, "SHUTTER_CLOSING_TIME"=w1668, "VERTICAL_SHIFT_SPEED"=w1667, "READ_MODE"=w1666, "VERTICAL_CLOCK_VOLTAGE"=w1665, "AD_CHANNEL"=w1664, "SHUTTER_MODE"=w1663, "SHUTTER_TTL"=w1662, "TRIGGER_MODE"=w1661, "FRAME_TRANSFER"=w1638, "ACQUISITION_MODE"=w1660, "EM_MODE"=w1659) -> (w1649:T24)
        n835 = call-dynamic "Set CCD_Config.vi"("error in (no error)"=w1679, "input cluster"=w1649, "Interface in"=w1680) -> ("error out"=w1684:errorcluster, "Interface out"=w1685:refnum<class "Interface.lvclass">)  [unwired: 7 in]
        n836 = Flatten To String(anything=w1649, error in (no error)=w1684) -> (data string=w1687:string, error out=w1686:errorcluster)  [unwired: 2 in, 1 out]
        n837 = call "Write flatted cluster.vi"("error in (no error)"=w1686, "flatted cluster"=w1687, "Interface in"=w1685) -> ("error out"=w1683:errorcluster, "Interface out"=w1682:refnum<class "Interface.lvclass">)  [unwired: 7 in]
        n838 = call-dynamic "Write Interface.vi"("error in (no error)"=w1683, "Interface.lvclass"=w1682, "Channel in"=w1700) -> ("error out"=w1654:errorcluster, "Channel out"=w1657:refnum<class "Channel.lvclass">)  [unwired: 7 in]
        n839 = call "Write section_name.vi"("error in (no error)"=w1654, "section_name"="CCD_ACS2", "Channel in"=w1657) -> ("error out"=w1653:errorcluster, "Channel out"=w1656:refnum<class "Channel.lvclass">)  [unwired: 7 in]
        n840 = call-dynamic "save config.vi"("error in (no error)"=w1653, "file config"="lastsaved.cfg", "Channel in"=w1656) -> ("error out"=w1652:errorcluster, "Channel out"=w1655:refnum<class "Channel.lvclass">)  [unwired: 7 in]
        n841 = call-dynamic "Read State Machine.vi"("error in (no error)"=w1652, "Device in"=w1655) -> ("error out"=w1694:errorcluster, "State Machine.lvclass"=w1696:refnum<class "State Machine.lvclass">, "Device out"=w1697:refnum<class "Channel.lvclass">)  [unwired: 7 in]
        n842 = call-dynamic "Write State.vi"("error in (no error)"=w1694, "State"=60, "State Machine in"=w1696) -> ("error out"=w1693:errorcluster, "State Machine out"=w1695:refnum<class "State Machine.lvclass">)  [unwired: 7 in]
        n843 = call-dynamic "Write State Machine.vi"("error in (no error)"=w1693, "State Machine.lvclass"=w1695, "Device in"=w1697) -> ("error out"=w1690:errorcluster, "Device out"=w1691:refnum<class "Channel.lvclass">)  [unwired: 7 in]
        n844 = call-dynamic "Write Channel.vi"("error in (no error)"=w1690, "Channel.lvclass"=w1691, "Acquisition in"=w1702) -> ("error out"=w1689:errorcluster, "Acquisition out"=w1688:refnum<class "Acquisition.lvclass">)  [unwired: 7 in]
        n845 = call "Write AcquisitionB.vi"("error in (no error)"=w1689, "Acquisition.lvclass"=w1688, "S4ACS_GUI in"=w1704) -> ("error out"=w1643:errorcluster, "S4ACS_GUI out"=w1644:refnum<class "S4GUI.lvclass">)  [unwired: 7 in]
        n846 = call "Write cfg file.vi"("error in (no error)"=w1643, "cfg file"="lastsaved.cfg", "S4ACS_GUI in"=w1644) -> ("error out"=w1646:errorcluster, "S4ACS_GUI out"=w1647:refnum<class "S4GUI.lvclass">)  [unwired: 7 in]
      }
      event "Set from Input ch3": Value Change {
        n847 = event-data() -> ()  [unwired: 1 in, 6 out]
        n848 = local read "Input Cluster"() -> (w1720:T6)
        n849 = Unbundle By Name(w1720) -> ("Parameters"=w1719:T23)
        n850 = Unbundle By Name(w1719) -> ("Image \nInitial Line"=w1747:u16, "Image\nInitial Column"=w1746:u16, "Image\nFinal Line"=w1745:u16, "Image\nFInal Column"=w1744:u16, "Vertical\nBinning"=w1743:u16, "Horizontal\nBinning"=w1742:u16, "Pre-amplification\nGain"=w1741:u8, "CCD\nEM Gain"=w1740:u16, "Readout\nRate"=w1739:u8, "Shutter\nOpenning Time"=w1738:i32, "Shutter\nClosing Time"=w1737:i32, "Vertical\nShift Speed"=w1736:u8, "Read\nMode"=w1735:u8, "Vertical\nClock Voltage"=w1734:u8, "A/D \nChannel"=w1733:u32, "Shutter\nMode"=w1732:u16, "Shutter\nTTL"=w1731:u16, "Trigger\nMode"=w1730:u16, "Frame\nTransfer"=w1707:bool, "Acquisition\nMode"=w1729:u8, "CCD \nEM Mode"=w1728:u8)
        n851 = call-dynamic "Read AcquisitionC.vi"("error in (no error)"=w1774, "S4ACS_GUI in"=w1775) -> ("error out"=w1768:errorcluster, "Acquisition.lvclass"=w1772:refnum<class "Acquisition.lvclass">, "S4ACS_GUI out"=w1773:refnum<class "S4GUI.lvclass">)  [unwired: 7 in]
        n852 = call-dynamic "Read Channel.vi"("error in (no error)"=w1768, "Acquisition in"=w1772) -> ("error out"=w1767:errorcluster, "Channel.lvclass"=w1770:refnum<class "Channel.lvclass">, "Acquisition out"=w1771:refnum<class "Acquisition.lvclass">)  [unwired: 7 in]
        n853 = call-dynamic "Read Interface.vi"("error in (no error)"=w1767, "Channel in"=w1770) -> ("error out"=w1710:errorcluster, "Interface.lvclass"=w1711:refnum<class "Interface.lvclass">, "Channel out"=w1769:refnum<class "Channel.lvclass">)  [unwired: 7 in]
        n854 = call-dynamic "Write PREV_FT.vi"("error in (no error)"=w1710, "PREV_FT"=w1707, "Interface in"=w1711) -> ("error out"=w1708:errorcluster, "Interface out"=w1709:refnum<class "Interface.lvclass">)  [unwired: 7 in]
        n855 = call-dynamic "Get CCD_Config.vi"("error in (no error)"=w1708, "Interface in"=w1709) -> ("error out"=w1748:errorcluster, "output cluster"=w1750:T24, "Interface out"=w1749:refnum<class "Interface.lvclass">)  [unwired: 7 in]
        n856 = Bundle By Name(cluster=w1750, "INITIAL_LINE"=w1747, "INITIAL_COLUMN"=w1746, "FINAL_LINE"=w1745, "FINAL_COLUMN"=w1744, "VBIN"=w1743, "HBIN"=w1742, "PREAMP"=w1741, "EM_GAIN"=w1740, "READOUT_RATE"=w1739, "SHUTTER_OPENING_TIME"=w1738, "SHUTTER_CLOSING_TIME"=w1737, "VERTICAL_SHIFT_SPEED"=w1736, "READ_MODE"=w1735, "VERTICAL_CLOCK_VOLTAGE"=w1734, "AD_CHANNEL"=w1733, "SHUTTER_MODE"=w1732, "SHUTTER_TTL"=w1731, "TRIGGER_MODE"=w1730, "FRAME_TRANSFER"=w1707, "ACQUISITION_MODE"=w1729, "EM_MODE"=w1728) -> (w1718:T24)
        n857 = call-dynamic "Set CCD_Config.vi"("error in (no error)"=w1748, "input cluster"=w1718, "Interface in"=w1749) -> ("error out"=w1753:errorcluster, "Interface out"=w1754:refnum<class "Interface.lvclass">)  [unwired: 7 in]
        n858 = Flatten To String(anything=w1718, error in (no error)=w1753) -> (data string=w1756:string, error out=w1755:errorcluster)  [unwired: 2 in, 1 out]
        n859 = call "Write flatted cluster.vi"("error in (no error)"=w1755, "flatted cluster"=w1756, "Interface in"=w1754) -> ("error out"=w1752:errorcluster, "Interface out"=w1751:refnum<class "Interface.lvclass">)  [unwired: 7 in]
        n860 = call-dynamic "Write Interface.vi"("error in (no error)"=w1752, "Interface.lvclass"=w1751, "Channel in"=w1769) -> ("error out"=w1723:errorcluster, "Channel out"=w1726:refnum<class "Channel.lvclass">)  [unwired: 7 in]
        n861 = call "Write section_name.vi"("error in (no error)"=w1723, "section_name"="CCD_ACS3", "Channel in"=w1726) -> ("error out"=w1722:errorcluster, "Channel out"=w1725:refnum<class "Channel.lvclass">)  [unwired: 7 in]
        n862 = call-dynamic "save config.vi"("error in (no error)"=w1722, "file config"="lastsaved.cfg", "Channel in"=w1725) -> ("error out"=w1721:errorcluster, "Channel out"=w1724:refnum<class "Channel.lvclass">)  [unwired: 7 in]
        n863 = call-dynamic "Read State Machine.vi"("error in (no error)"=w1721, "Device in"=w1724) -> ("error out"=w1763:errorcluster, "State Machine.lvclass"=w1765:refnum<class "State Machine.lvclass">, "Device out"=w1766:refnum<class "Channel.lvclass">)  [unwired: 7 in]
        n864 = call-dynamic "Write State.vi"("error in (no error)"=w1763, "State"=60, "State Machine in"=w1765) -> ("error out"=w1762:errorcluster, "State Machine out"=w1764:refnum<class "State Machine.lvclass">)  [unwired: 7 in]
        n865 = call-dynamic "Write State Machine.vi"("error in (no error)"=w1762, "State Machine.lvclass"=w1764, "Device in"=w1766) -> ("error out"=w1759:errorcluster, "Device out"=w1760:refnum<class "Channel.lvclass">)  [unwired: 7 in]
        n866 = call-dynamic "Write Channel.vi"("error in (no error)"=w1759, "Channel.lvclass"=w1760, "Acquisition in"=w1771) -> ("error out"=w1758:errorcluster, "Acquisition out"=w1757:refnum<class "Acquisition.lvclass">)  [unwired: 7 in]
        n867 = call-dynamic "Write AcquisitionC.vi"("error in (no error)"=w1758, "Acquisition.lvclass"=w1757, "S4ACS_GUI in"=w1773) -> ("error out"=w1712:errorcluster, "S4ACS_GUI out"=w1713:refnum<class "S4GUI.lvclass">)  [unwired: 7 in]
        n868 = call "Write cfg file.vi"("error in (no error)"=w1712, "cfg file"="lastsaved.cfg", "S4ACS_GUI in"=w1713) -> ("error out"=w1715:errorcluster, "S4ACS_GUI out"=w1716:refnum<class "S4GUI.lvclass">)  [unwired: 7 in]
      }
      event "Set from Input ch4": Value Change {
        n869 = event-data() -> ()  [unwired: 1 in, 6 out]
        n870 = local read "Input Cluster"() -> (w1789:T6)
        n871 = Unbundle By Name(w1789) -> ("Parameters"=w1788:T23)
        n872 = Unbundle By Name(w1788) -> ("Image \nInitial Line"=w1816:u16, "Image\nInitial Column"=w1815:u16, "Image\nFinal Line"=w1814:u16, "Image\nFInal Column"=w1813:u16, "Vertical\nBinning"=w1812:u16, "Horizontal\nBinning"=w1811:u16, "Pre-amplification\nGain"=w1810:u8, "CCD\nEM Gain"=w1809:u16, "Readout\nRate"=w1808:u8, "Shutter\nOpenning Time"=w1807:i32, "Shutter\nClosing Time"=w1806:i32, "Vertical\nShift Speed"=w1805:u8, "Read\nMode"=w1804:u8, "Vertical\nClock Voltage"=w1803:u8, "A/D \nChannel"=w1802:u32, "Shutter\nMode"=w1801:u16, "Shutter\nTTL"=w1800:u16, "Trigger\nMode"=w1799:u16, "Frame\nTransfer"=w1776:bool, "Acquisition\nMode"=w1798:u8, "CCD \nEM Mode"=w1797:u8)
        n873 = call-dynamic "Read AcquisitionD.vi"("error in (no error)"=w1843, "S4ACS_GUI in"=w1844) -> ("error out"=w1837:errorcluster, "Acquisition.lvclass"=w1841:refnum<class "Acquisition.lvclass">, "S4ACS_GUI out"=w1842:refnum<class "S4GUI.lvclass">)  [unwired: 7 in]
        n874 = call-dynamic "Read Channel.vi"("error in (no error)"=w1837, "Acquisition in"=w1841) -> ("error out"=w1836:errorcluster, "Channel.lvclass"=w1839:refnum<class "Channel.lvclass">, "Acquisition out"=w1840:refnum<class "Acquisition.lvclass">)  [unwired: 7 in]
        n875 = call-dynamic "Read Interface.vi"("error in (no error)"=w1836, "Channel in"=w1839) -> ("error out"=w1779:errorcluster, "Interface.lvclass"=w1780:refnum<class "Interface.lvclass">, "Channel out"=w1838:refnum<class "Channel.lvclass">)  [unwired: 7 in]
